vi "Add Customer.vi"(8 "error in (no error)":errorcluster, 11 "Coffee Shop in":refnum<class "Coffee Shop.lvclass">) -> (0 "error out":errorcluster, 3 "Coffee Shop out":refnum<class "Coffee Shop.lvclass">)   [LabVIEW 2023, in "Coffee Shop.lvlib" / "Coffee Shop.lvclass"]
doc: "Instantiate a new Customer actor"
uses:
  Coffee Shop.lvclass
  c:/dev/_r/4/eng/lv-core/lvpostprocessingd/lv_mc_x86_64/dist_i386/vi.lib/ActorFramework/Actor/Actor.lvclass
  Customer/Children/CustomerWithCellPhone/Customer With Cell Phone.lvclass
  Coffee Shop.lvclass/Coffee Shop.ctl
  Entity Table/Entity Data.ctl
  Entity Types.ctl
  Entity Table/Entity Table.lvclass
  <vilib>/ActorFramework/Actor/Actor.lvclass
panel:
  in  "Reading menu":string="Reading menu..."
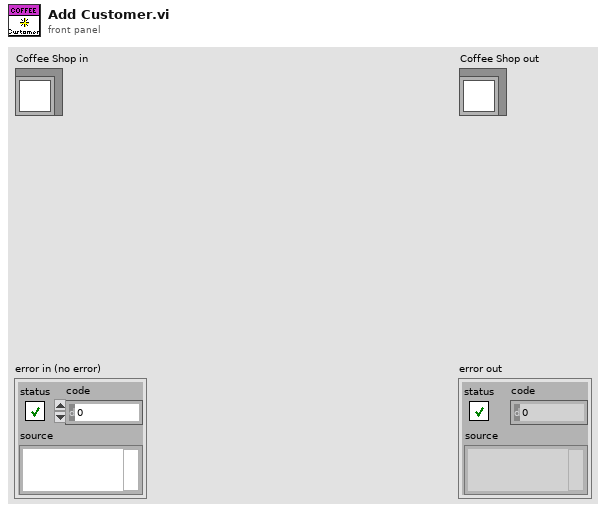
[diagram p1: front panel]
types:
  T1 = typedef "Coffee Shop.lvlib/Coffee Shop.lvclass/Entity Types.ctl" = enum16{"Customer", "Cashier", "Barista"}
  T2 = typedef "Entity Table.lvclass/Entity Data.ctl" = cluster{"Name":string, "Status":string}
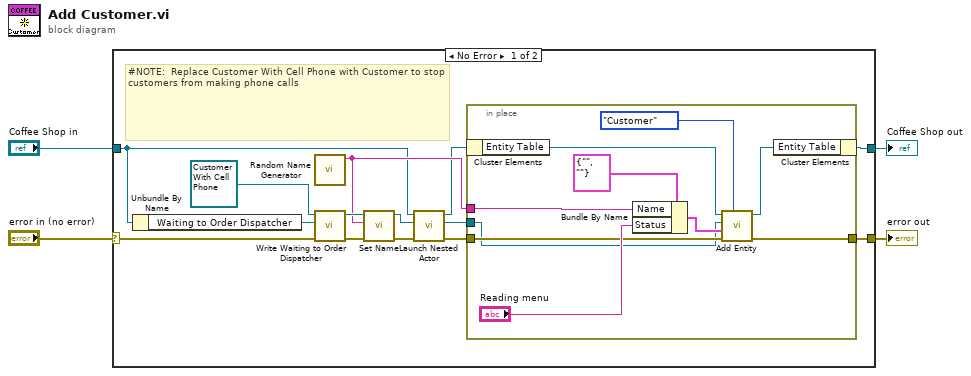
[diagram p0: block diagram]
diagram:
  n1 = case shown="No Error" "error in (no error)" {
    selector: "error in (no error)" -> [w16 w30]
    tunnel: [w9 w30] -> w3
    tunnel: [w18 w29] -> w1
    tunnel: "Coffee Shop in" -> [w6 w29]
    frame No Error {
      # "#NOTE:  Replace Customer With Cell Phone with Customer to stop customers from making phone calls"
      n2 = Unbundle By Name(w6) -> ("Waiting to Order Dispatcher"=w15:refnum<class "Message Enqueuer.lvclass">)
      n3 = call "Random Name Generator.vi"() -> ("Name"=w10:string)  [unwired: 11 in]
      n4 = call-dynamic "Write Waiting to Order Dispatcher.vi"("error in (no error)"=w16, "Actor Framework.lvlib:Message Enqueuer"=w15, "Customer in"=refnum<class "Customer With Cell Phone.lvclass"> refnum ("CustomerWithCellPhone.lvlib:CustomerWithCellPhone.lvclass")) -> ("error out"=w13:errorcluster, "Customer out"=w11:refnum<class "Customer With Cell Phone.lvclass">)  [unwired: 7 in]
      n5 = call-dynamic "Set Name.vi"("error in (no error)"=w13, "Name"=w10, "Person in"=w11) -> ("error out"=w12:errorcluster, "Person out"=w7:refnum<class "Customer With Cell Phone.lvclass">)  [unwired: 7 in]
      n6 = call <vilib>:"Launch Nested Actor.vi"("error in (no error)"=w12, "Nested Actor"=w7, "Caller Actor in"=w6) -> ("error out"=w14:errorcluster, "Nested Actor's Enqueuer"=w17:refnum<class "Message Enqueuer.lvclass">, "Caller Actor out"=w5:refnum<class "Coffee Shop.lvclass">)  [unwired: 6 in]
      n7 = in-place "In Place Element Structure" {
        in-place-border: w17 -> [w20]
        in-place-border: w14 -> [w21]
        in-place-border: w10 -> [w27]
        in-place-border: [w25] -> w9
        n8 = in-place-cluster #1 ("Unbundle / Bundle Elements")(w5) -> ("Entity Table"=w23:refnum<class "Entity Table.lvclass">)
        n9 = Bundle By Name(cluster=T2 {"Name"="", "Status"=""} ("Entity"), "Name"=w27, "Status"="Reading menu") -> (w22:T2)
        n10 = call "Add Entity.vi"("entity type"=Entity_Types."Customer", "error in (no error)"=w21, "entity details"=w22, "enqueuer"=w20, "Entity Table in"=w23) -> ("error out"=w25:errorcluster, "Entity Table out"=w24:refnum<class "Entity Table.lvclass">)  [unwired: 5 in]
        n11 = in-place-cluster #1 ("Unbundle / Bundle Elements")("Entity Table"=w24) -> (w18:refnum<class "Coffee Shop.lvclass">)
      }
    }
    frame Error {
    }
  }
  "error out" <- w3
  "Coffee Shop out" <- w1
